vi "ProcessData.vi"(8 "error in (no error)":errorcluster, 9 "State":T1, 10 "Analog Data":T3, 11 "WhiteNoiseOrientationDetection in":refnum<class "WhiteNoiseOrientationDetection.lvclass">) -> (0 "error out":errorcluster, 1 "Fixated":bool, 2 "Trigger":T2=enum."Broke Fixation", 3 "WhiteNoiseOrientationDetection out":refnum<class "WhiteNoiseOrientationDetection.lvclass">)   [LabVIEW 2014, in "WhiteNoiseOrientationDetection.lvclass"]
uses:
  WhiteNoiseOrientationDetection.lvclass
  Core SubVIs/Controls/TYPE - Analog Data.ctl
  Trial Based Experiment Statechart/Trial Based Experiment.lvsc/Trigger.ctl
  Trial Based Experiment Statechart/Trial Based Experiment.lvsc/State.ctl
  WhiteNoiseOrientationDetection.lvclass/WhiteNoiseOrientationDetection.ctl
  <vilib>/measure/madcrms.llb/Basic Averaged DC-RMS for 1 Chan.vi
  Trial Based Experiment Statechart/Trial Based Experiment.lvsc
  Core SubVIs/Core SubVIs.lvlib
  <vilib>/measure/NI_MAPro.lvlib
  Acquisition/BehaviorData/BehaviorData.lvclass
panel:
  in  "Adjustment Rate":dbl=0.02
  in  "Toggle Fixation":bool
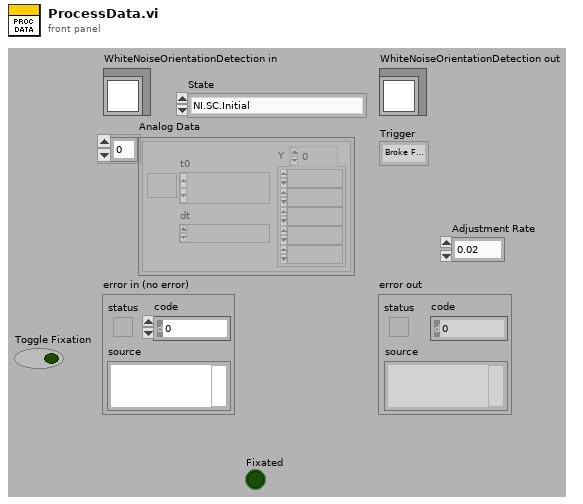
[diagram p1: front panel]
types:
  T1 = typedef "Trial Based Experiment.lvsc/State.ctl" = enum16{"NI.SC.Initial", "NI.SC.History", "NI.SC.ShallowHistory", "NI.SC.Terminal", "Cleanup", "State", "State\\Region\\Pause", "State\\Region\\Response Period", "State\\Region\\Delay Period", "State\\Region\\Hold Fixation", "State\\Region\\Acquire Fixation", "State\\Region\\Abort Trial", "State\\Region\\End Trial", "State\\Region\\Intertrial", "State\\Region\\Start Trial"}
  T2 = typedef "Trial Based Experiment.lvsc/Trigger.ctl" = enum16{"NULL", "Fixated", "Broke Fixation", "Stop", "Correct Response", "Incorrect Response", "Timeout"}
  T3 = typedef "Core SubVIs.lvlib/TYPE - Analog Data.ctl" = waveform(dbl)[]
  T4 = enum16{"Get Time", "Get Elapsed Time", "Reset Elapsed Time"}
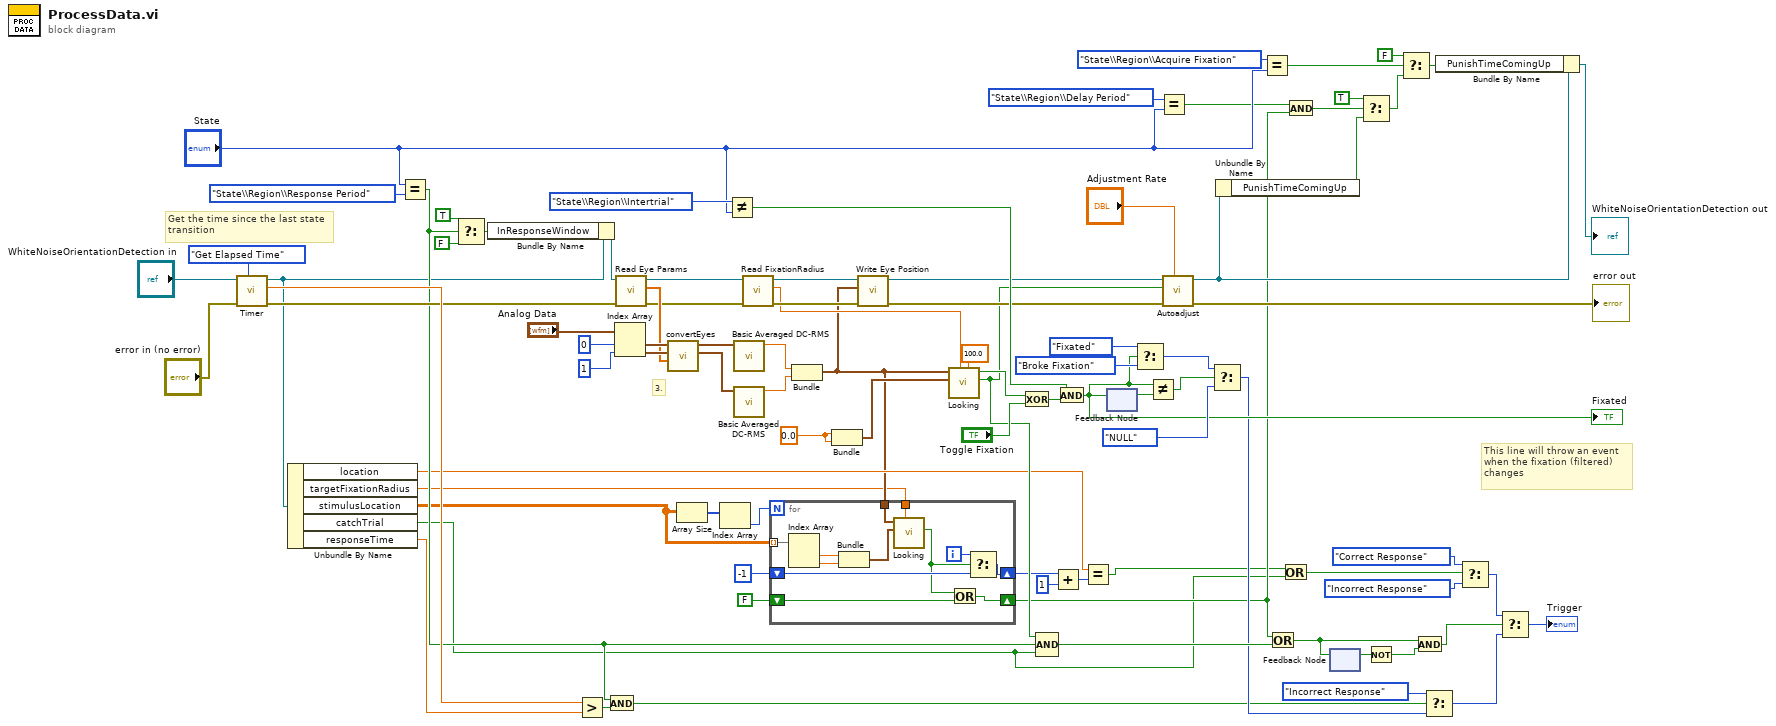
[diagram p0: block diagram]
diagram:
  w75 = 0.0
  # "Get the time since the last state\ntransition"
  # "This line will throw an event\nwhen the fixation (filtered)\nchanges"
  # "3."
  n1 = call-dynamic "Timer.vi"("Method"=T4."Get Elapsed Time", "error in (no error)"="error in (no error)", "BehaviorData in"="WhiteNoiseOrientationDetection in") -> ("error out"=w38:errorcluster, "Time"=w49:dbl, "BehaviorData out"=w21:refnum<class "WhiteNoiseOrientationDetection.lvclass">)  [unwired: 5 in, 1 out]
  n2 = Unbundle By Name(w21) -> ("location"=w14:dbl, "targetFixationRadius"=w5:dbl, "stimulusLocation"=w1:dbl[][], "catchTrial"=w2:bool, "responseTime"=w48:dbl)
  n3 = Equal?(x="State", y=State."State\\Region\\Response Period") -> (x = y?=w23:bool)
  n4 = Select(t=TRUE, s=w23, f=FALSE) -> (s? t:f=w19:bool)
  n5 = Bundle By Name(cluster=w21, "InResponseWindow"=w19) -> (w20:refnum<class "WhiteNoiseOrientationDetection.lvclass">)
  n6 = Greater?(x=w49, y=w48) -> (0:w45:bool)
  n7 = And(x=w23, y=w45) -> (x .and. y?=w44:bool)
  n8 = Index Array(array="Analog Data", index #1=0 ("index"), index #2=1 ("index")) -> (element #1=w89:waveform(dbl), element #2=w88:waveform(dbl))
  n9 = call-dynamic "Read Eye Params.vi"("error in (no error)"=w38, "TrialBasedExperiment in"=w20) -> ("error out"=w72:errorcluster, "Eye Params"=w80:dbl[], "TrialBasedExperiment out"=w39:refnum<class "WhiteNoiseOrientationDetection.lvclass">)  [unwired: 7 in]
  n10 = call "convertEyes.vi"("Params"=w80, "Vertical"=w88, "Horizontal"=w89) -> ("Vertical Calibrated"=w86:waveform(dbl), "Horizontal Calibrated"=w87:waveform(dbl))  [unwired: 7 in]
  n11 = Array Size(array=w1) -> (size(s)=w18:i32[])
  n12 = Index Array(array=w18) -> (element=w17:i32)  [unwired: 1 in]
  n13 = Not Equal?(x=State."State\\Region\\Intertrial", y="State") -> (x != y?=w66:bool)
  n14 = call-poly <vilib>:"Basic Averaged DC-RMS.vi"("signal in"=w87) -> ("DC value"=w78:dbl)  [unwired: 7 in, 3 out]
  n15 = call-poly <vilib>:"Basic Averaged DC-RMS.vi"("signal in"=w86) -> ("DC value"=w77:dbl)  [unwired: 7 in, 3 out]
  n16 = call-dynamic "Read FixationRadius.vi"("error in (no error)"=w72, "MatlabExperiment in"=w39) -> ("error out"=w70:errorcluster, "FixationRadius"=w69:dbl, "MatlabExperiment out"=w71:refnum<class "WhiteNoiseOrientationDetection.lvclass">)  [unwired: 7 in]
  n17 = Bundle("DC value"=w78, "DC value"=w77) -> (w6:cluster{"DC value":dbl, "DC value":dbl})  [unwired: 1 in]
  n18 = for {
    N: w17 -> [_]
    tunnel: w1 -> [w100] mode=indexing
    tunnel: w6 -> [w99]
    tunnel: w5 -> [w98]
    shift-right: [w97] -> w11
    shift-left: FALSE -> [w96]
    shift-right: [w94] -> w8
    shift-left: -1 -> [w93]
    i -> [w95]
    n19 = Index Array(array=w100) -> (element #1=w102:dbl, element #2=w101:dbl)  [unwired: 2 in]
    n20 = Bundle("Numeric"=w102, "Numeric"=w101) -> (w92:cluster{"Numeric":dbl, "Numeric":dbl})  [unwired: 1 in]
    n21 = call "Looking.vi"("Fixation Radius (px)"=w98, "Desired Position"=w92, "Eye Position"=w99) -> ("Looking Unfiltered"=w91:bool)  [unwired: 7 in, 1 out]
    n22 = Or(x=w91, y=w96) -> (x .or. y?=w97:bool)
    n23 = Select(t=w95, s=w91, f=w93) -> (s? t:f=w94:i32)
  }
  n24 = Bundle(w75, w75) -> (w76:cluster{dbl, dbl})  [unwired: 1 in]
  n25 = call-dynamic "Write Eye Position.vi"("error in (no error)"=w70, "Eye Position"=w6, "TrialBasedExperiment in"=w71) -> ("error out"=w62:errorcluster, "TrialBasedExperiment out"=w63:refnum<class "WhiteNoiseOrientationDetection.lvclass">)  [unwired: 7 in]
  n26 = call "Looking.vi"("Break Timeout (ms)"=100.0 ("f"), "Fixation Radius (px)"=w69, "Desired Position"=w76, "Eye Position"=w6) -> ("Looking Unfiltered"=w51:bool, "Looking"=w73:bool)  [unwired: 6 in]
  n27 = Exclusive Or(1:"Toggle Fixation", 2:w73) -> (0:w67:bool)
  n28 = Compound Arithmetic op=AND(w51, w23, w2) -> (w50:bool)
  n29 = Add(x=w8, y=1) -> (x+y=w9:i32)
  n30 = And(x=w66, y=w67) -> (x .and. y?=w55:bool)
  "Fixated" <- w55
  n31 = Equal?(x=w14, y=w9) -> (x = y?=w3:bool)
  n32 = feedback #1() -> (w85:bool)  [unwired: 1 in]
  n33 = feedback-in #1(w55) -> ()
  n34 = Select(t=Trigger."Fixated" ("Trigger"), s=w55, f=Trigger."Broke Fixation" ("Trigger")) -> (s? t:f=w83:T2)
  n35 = Not Equal?(x=w55, y=w85) -> (x != y?=w64:bool)
  n36 = Equal?(x=State."State\\Region\\Delay Period" ("y"), y="State") -> (x = y?=w28:bool)
  n37 = call-dynamic "Autoadjust.vi"("Adjustment Rate"="Adjustment Rate", "error in (no error)"=w62, "Fixated"=w51, "TrialBasedExperiment in"=w63) -> ("error out"=→"error out":errorcluster, "TrialBasedExperiment out"=w26:refnum<class "WhiteNoiseOrientationDetection.lvclass">)  [unwired: 6 in]
  n38 = Select(t=w83, s=w64, f=Trigger."NULL" ("Trigger")) -> (s? t:f=w46:T2)
  n39 = Unbundle By Name(w26) -> ("PunishTimeComingUp"=w25:bool)
  n40 = Equal?(x=State."State\\Region\\Acquire Fixation" ("y"), y="State") -> (x = y?=w36:bool)
  n41 = Or(x=w11, y=w50) -> (x .or. y?=w41:bool)
  n42 = Or(x=w3, y=w2) -> (x .or. y?=w4:bool)
  n43 = And(x=w28, y=w11) -> (x .and. y?=w29:bool)
  n44 = feedback-in #2(w41) -> ()
  n45 = feedback #2() -> (w43:bool)  [unwired: 1 in]
  n46 = Select(t=TRUE, s=w29, f=w25) -> (s? t:f=w33:bool)
  n47 = Not(x=w43) -> (.not. x?=w42:bool)
  n48 = Select(t=FALSE, s=w36, f=w33) -> (s? t:f=w34:bool)
  n49 = And(x=w41, y=w42) -> (x .and. y?=w40:bool)
  n50 = Select(t=Trigger."Incorrect Response", s=w44, f=w46) -> (s? t:f=w53:T2)
  n51 = Bundle By Name(cluster=w26, "PunishTimeComingUp"=w34) -> (→"WhiteNoiseOrientationDetection out":refnum<class "WhiteNoiseOrientationDetection.lvclass">)
  n52 = Select(t=Trigger."Correct Response", s=w4, f=Trigger."Incorrect Response" ("t")) -> (s? t:f=w10:T2)
  n53 = Select(t=w10, s=w40, f=w53) -> (s? t:f=→"Trigger":T2)
